vi "Wait on Listener.vi"(0 "Listener ID in":refnum<k5>[](array[refnum]), 5 "ETH_Names":string[](array[string])) -> (4 "Connection ID":refnum<k5>[](array[refnum]), 6 "Listener ID":refnum<k5>[](array[refnum]), 8 "Connected":string[](array[string]), 10 "Not connected":string[](array[string]), 15 "Status":bool[](array[boolean]))   [LabVIEW 2022 SP3]
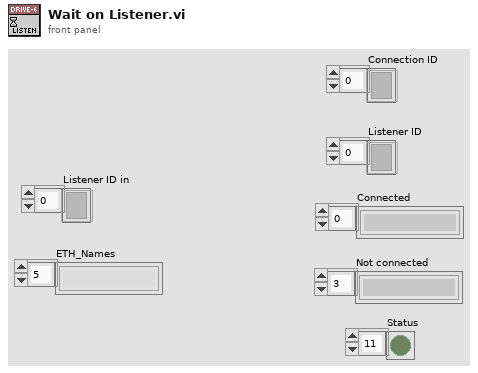
[diagram p1: front panel]
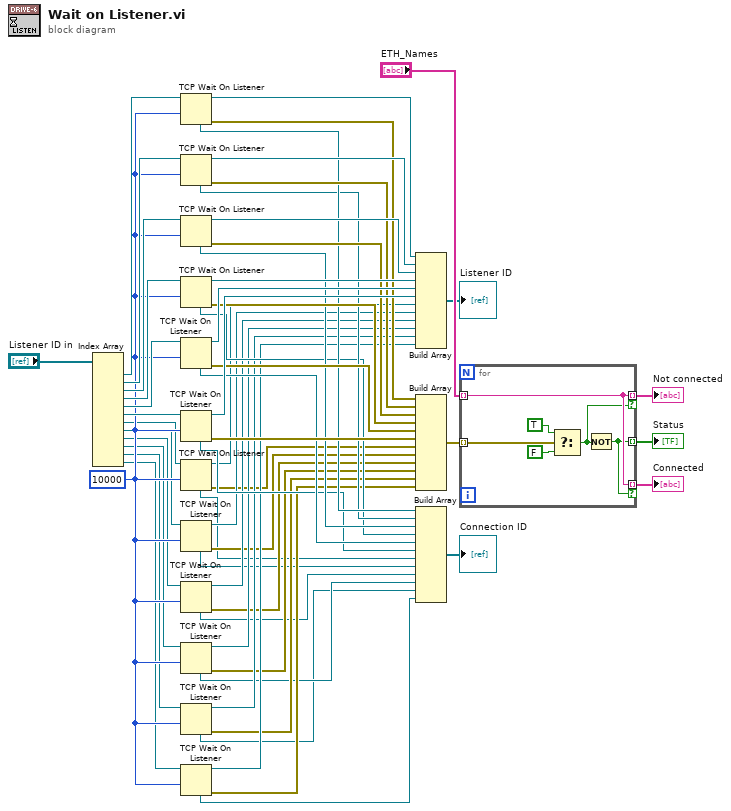
[diagram p0: block diagram]
diagram:
  w25 = 10000 ("timeout ms (wait forever: -1)")
  n1 = Index Array(array="Listener ID in") -> (element #1=w56:refnum<k5>, element #2=w55:refnum<k5>, element #3=w54:refnum<k5>, element #4=w53:refnum<k5>, element #5=w52:refnum<k5>, element #6=w51:refnum<k5>, element #7=w24:refnum<k5>, element #8=w23:refnum<k5>, element #9=w22:refnum<k5>, element #10=w21:refnum<k5>, element #11=w20:refnum<k5>, element #12=w19:refnum<k5>)  [unwired: 12 in]
  n2 = TCP Wait On Listener(9:w25, 11:w56) -> (0:w44:errorcluster, 3:w50:refnum<k5>, 4:w33:refnum<k5>)  [unwired: 1 in, 3 out]
  n3 = TCP Wait On Listener(9:w25, 11:w55) -> (0:w43:errorcluster, 3:w49:refnum<k5>, 4:w32:refnum<k5>)  [unwired: 2 in, 2 out]
  n4 = TCP Wait On Listener(9:w25, 11:w54) -> (0:w42:errorcluster, 3:w48:refnum<k5>, 4:w31:refnum<k5>)  [unwired: 1 in, 3 out]
  n5 = TCP Wait On Listener(9:w25, 11:w53) -> (0:w41:errorcluster, 3:w47:refnum<k5>, 4:w30:refnum<k5>)  [unwired: 1 in, 3 out]
  n6 = TCP Wait On Listener(9:w25, 11:w52) -> (0:w40:errorcluster, 3:w46:refnum<k5>, 4:w29:refnum<k5>)  [unwired: 1 in, 3 out]
  n7 = TCP Wait On Listener(9:w25, 11:w51) -> (0:w39:errorcluster, 3:w45:refnum<k5>, 4:w28:refnum<k5>)  [unwired: 1 in, 3 out]
  n8 = TCP Wait On Listener(9:w25, 11:w24) -> (0:w12:errorcluster, 3:w18:refnum<k5>, 4:w6:refnum<k5>)  [unwired: 1 in, 3 out]
  n9 = TCP Wait On Listener(9:w25, 11:w23) -> (0:w11:errorcluster, 3:w17:refnum<k5>, 4:w5:refnum<k5>)  [unwired: 2 in, 2 out]
  n10 = TCP Wait On Listener(9:w25, 11:w22) -> (0:w10:errorcluster, 3:w16:refnum<k5>, 4:w4:refnum<k5>)  [unwired: 1 in, 3 out]
  n11 = TCP Wait On Listener(9:w25, 11:w21) -> (0:w9:errorcluster, 3:w15:refnum<k5>, 4:w3:refnum<k5>)  [unwired: 1 in, 3 out]
  n12 = TCP Wait On Listener(9:w25, 11:w20) -> (0:w8:errorcluster, 3:w14:refnum<k5>, 4:w2:refnum<k5>)  [unwired: 1 in, 3 out]
  n13 = TCP Wait On Listener(9:w25, 11:w19) -> (0:w7:errorcluster, 3:w13:refnum<k5>, 4:w1:refnum<k5>)  [unwired: 1 in, 3 out]
  n14 = Build Array(w50, w49, w48, w47, w46, w45, w18, w17, w16, w15, w14, w13) -> (→"Listener ID":refnum<k5>[])
  n15 = Build Array(w44, w43, w42, w41, w40, w39, w12, w11, w10, w9, w8, w7) -> (w34:errorcluster[])
  n16 = Build Array(w33, w32, w31, w30, w29, w28, w6, w5, w4, w3, w2, w1) -> (→"Connection ID":refnum<k5>[])
  n17 = for {
    tunnel: w34 -> [w62] mode=indexing
    tunnel: "ETH_Names" -> [w63] mode=indexing
    tunnel: [w63] -> w37 mode=indexing if=w58
    tunnel: [w63] -> w36 mode=indexing if=w59
    tunnel: [w58] -> w35 mode=indexing
    n18 = Select(t=TRUE, s=w62, f=FALSE) -> (s? t:f=w59:bool)
    n19 = Not(x=w59) -> (.not. x?=w58:bool)
  }
  "Connected" <- w37
  "Not connected" <- w36
  "Status" <- w35
